vi "Test_Observe_ViewablePublication_OK.vi"(8 "error in (no error)":errorcluster, 11 "TestObservation In":refnum<class "TestObservation.lvclass">) -> (0 "error out":errorcluster, 3 "TestObservation Out":refnum<class "TestObservation.lvclass">)   [LabVIEW 2015, in "TestObservation.lvclass"]
uses:
  TestObservation.lvclass
  Framework/Mediator/Mediator/Mediator.lvclass
  PublishingViewable/PublishingViewable.lvclass
  Framework/IViewModel/IViewModel/IViewModel.lvclass/IViewModel.ctl
  Framework/IViewManager/IViewManager Messages/Launch Nested Views Msg/Launch Nested Views Msg.lvclass/Launch Nested Views Msg.ctl
  Framework/IViewManager/IViewManager/IViewManager.lvclass/IViewManager.ctl
  <vilib>/ActorFramework/Message Enqueuer/Message Enqueuer.lvclass/Message Enqueuer.ctl
  Framework/IViewManager/IViewManager Messages/Launch Nested Views Msg/Pack Launch Nested Views Msg.vi
  Framework/IViewManager/IViewManager/Write Startup Launch Nested Views Msg.vi
  <vilib>/ActorFramework/Message Enqueuer/Enqueue.vi
  <vilib>/ActorFramework/Message Priority Queue/Priority Enqueue.vi
  Framework/IViewable/IApplicationStyle/IApplicationStyle.lvclass
  Framework/IViewManager/IViewManager Messages/Launch Nested Views Msg/Launch Nested Views Msg.lvclass
  <vilib>/ActorFramework/Stop Msg/Stop Msg.lvclass
  <vilib>/addons/_JKI Toolkits/VI Tester/TestCase.llb/TestCase.lvclass
  Framework/IViewModel/IViewModel/IViewModel.lvclass
  <vilib>/ActorFramework/Actor/Actor.lvclass
  ObservingModel/ObservingModel.lvclass
  ObservingViewModel/ObservingViewModel.lvclass
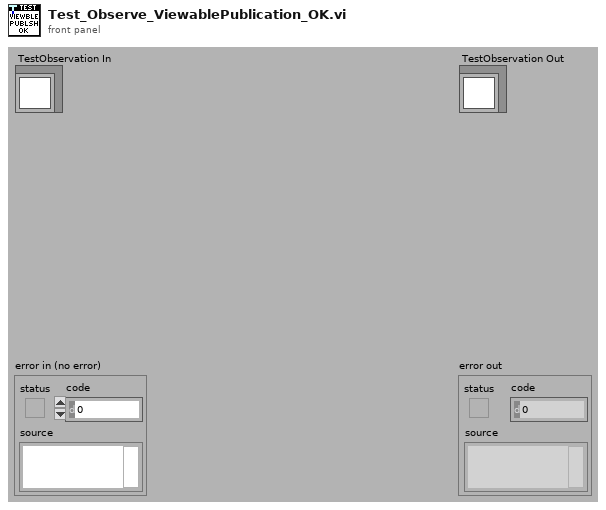
[diagram p1: front panel]
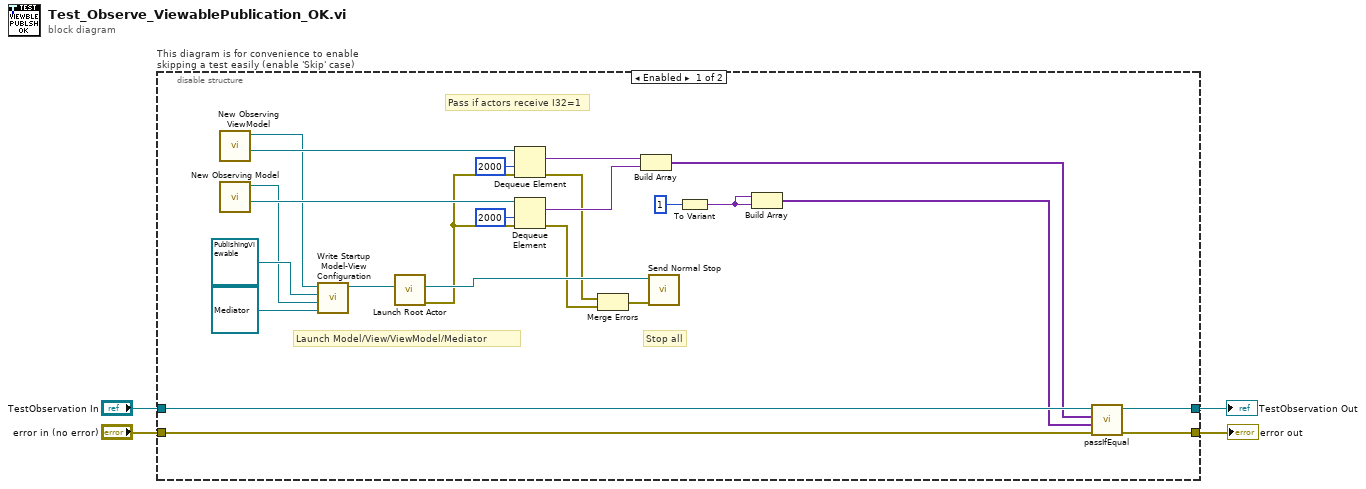
[diagram p0: block diagram]
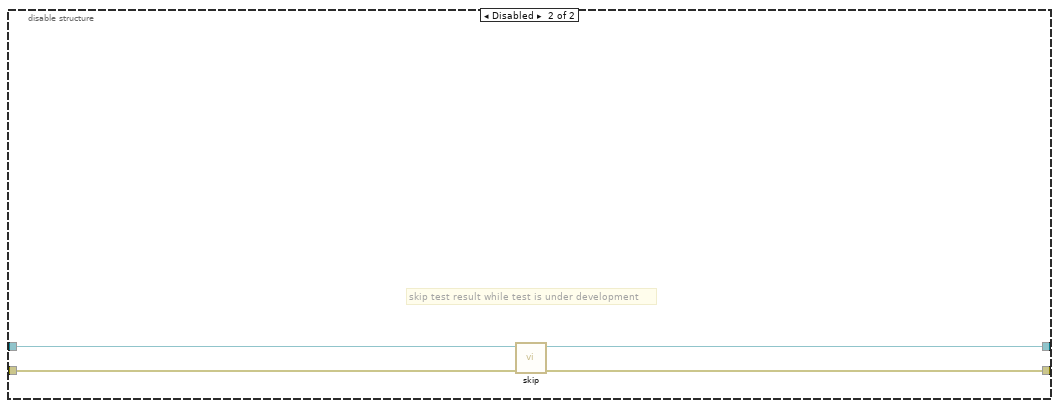
[diagram p2: hidden frame]
diagram:
  n1 = disable-structure "This diagram is for convenience to enable skipping a test easily (enable 'Skip' case)" shown="Enabled" {
    disable-tunnel: "TestObservation In" -> [w28 w32]
    disable-tunnel: [w27 w30] -> w1
    disable-tunnel: [w26 w31] -> w3
    disable-tunnel: "error in (no error)" -> [w25 w29]
    frame Enabled {
      # "Stop all"
      # "Launch Model/View/ViewModel/Mediator"
      # "Pass if actors receive I32=1"
      n2 = call "New Observing ViewModel.vi"() -> ("Test Reply Queue"=w14:refnum<queue>, "ObservingViewModel Out"=w9:refnum<class "ObservingViewModel.lvclass">)  [unwired: 10 in]
      n3 = call "New Observing Model.vi"() -> ("Test Reply Queue"=w17:refnum<queue>, "ObservingModel Out"=w10:refnum<class "ObservingModel.lvclass">)  [unwired: 10 in]
      n4 = call "Write Startup Model-View Configuration.vi"("Mediator Type"=refnum<class "Mediator.lvclass"> refnum ("Mediator.lvlib:Mediator.lvclass"), "Model Type"=w10, "Startup View Configuration"=refnum<class "PublishingViewable.lvclass"> refnum ("PublishingViewable.lvclass"), "IViewModel In"=w9) -> ("IViewModel Out"=w23:refnum<class "ObservingViewModel.lvclass">)  [unwired: 7 in]
      n5 = call <vilib>:"Launch Root Actor.vi"("Actor"=w23) -> ("error out"=w13:errorcluster, "Actor's Enqueuer"=w21:refnum<class "Message Enqueuer.lvclass">)  [unwired: 9 in]
      n6 = Dequeue Element(queue=w14, timeout in ms (-1)=2000, error in (no error)=w13) -> (element=w7:variant, error out=w11:errorcluster)  [unwired: 2 out]
      n7 = Dequeue Element(queue=w17, timeout in ms (-1)=2000, error in (no error)=w13) -> (element=w19:variant, error out=w20:errorcluster)  [unwired: 2 out]
      n8 = Merge Errors(w11, w20) -> (w12:errorcluster)
      n9 = Build Array(w7, w19) -> (w8:variant[])
      n10 = call <vilib>:"Send Normal Stop.vi"("error in (no error)"=w12, "Message Enqueuer"=w21) -> ()  [unwired: 9 in, 1 out]
      n11 = To Variant(anything=1) -> (Variant=w5:variant)
      n12 = Build Array(w5, w5) -> (w6:variant[])
      n13 = call-dynamic "passIfEqual.vi"("error in (no error)"=w25, "y"=w6, "x"=w8, "TestCase in"=w28) -> ("error out"=w26:errorcluster, "TestCase out"=w27:refnum<class "TestObservation.lvclass">)  [unwired: 6 in]
    }
    frame Disabled {
      # "skip test result while test is under development"
      n14 = call <vilib>:"skip.vi"("error in (no error)"=w29, "TestCase in"=w32) -> ("error out"=w31:errorcluster, "TestCase out"=w30:refnum<class "TestObservation.lvclass">)  [unwired: 8 in]
    }
  }
  "error out" <- w3
  "TestObservation Out" <- w1
